vi "DHE_set_roi_transf.vi"(8 "error in (no error)":errorcluster, 10 "args":string) -> (0 "error out":errorcluster, 1 "full":bool, 2 "roi":string, 4 "add roi":bool)   [LabVIEW 2016]
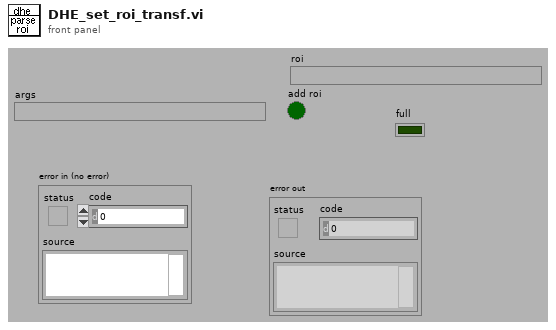
[diagram p1: front panel]
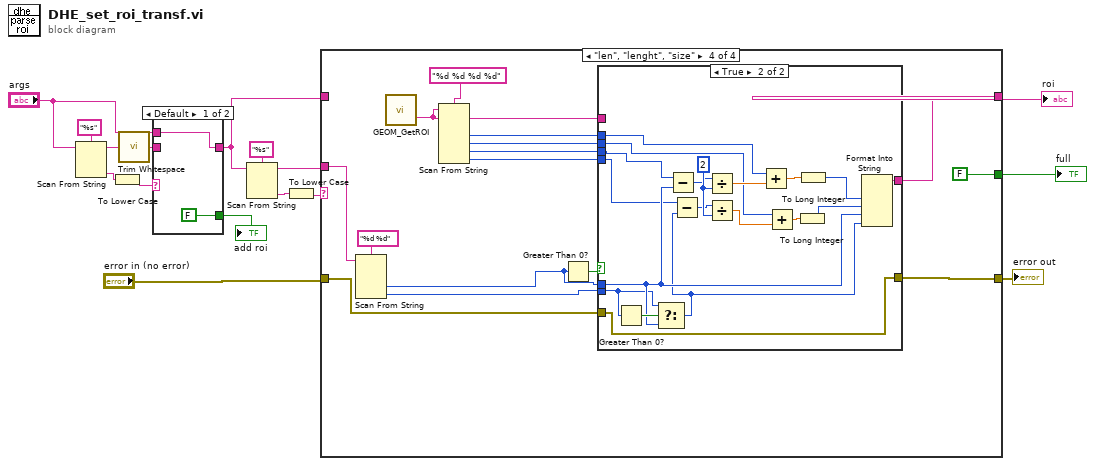
[diagram p0: block diagram]
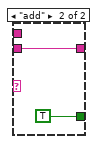
[diagram p2: hidden frame]
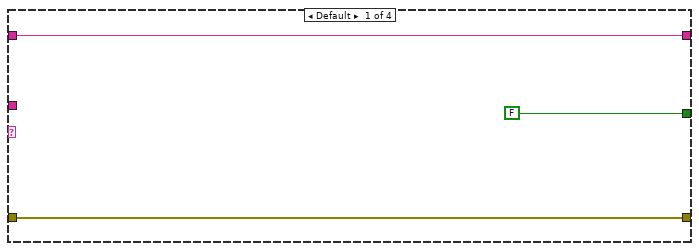
[diagram p3: hidden frame]
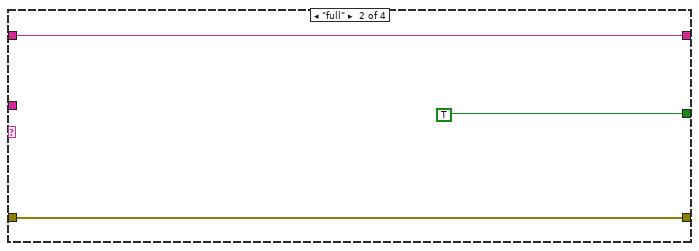
[diagram p4: hidden frame]
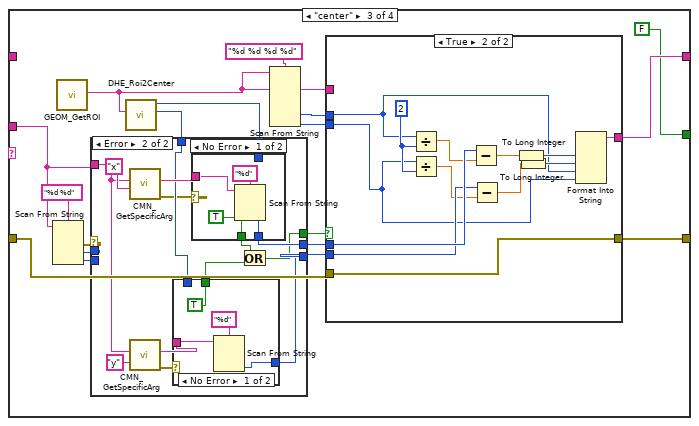
[diagram p5: hidden frame]
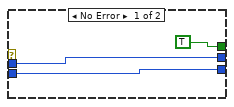
[diagram p6: hidden frame]
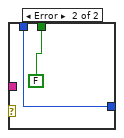
[diagram p7: hidden frame]
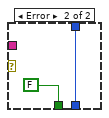
[diagram p8: hidden frame]
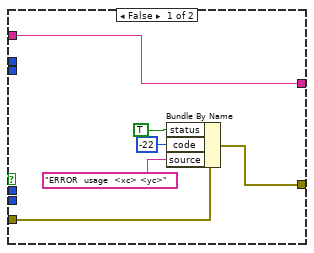
[diagram p9: hidden frame]
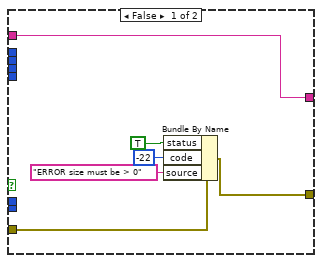
[diagram p10: hidden frame]
diagram:
  n1 = Scan From String(format string="%s", input string="args") -> (remaining string=w5:string, output 1=w7:string)  [unwired: 2 in, 3 out]
  n2 = To Lower Case(string=w7) -> (all lower case string=w6:string)
  n3 = call <vilib>:"Trim Whitespace.vi"("string"=w5) -> ("trimmed string"=w4:string)  [unwired: 1 in]
  n4 = case shown="Default" w6 {
    tunnel: w4 -> [_ w20]
    tunnel: [w18 w20] -> w3
    tunnel: "args" -> [w18 _]
    tunnel: [FALSE TRUE] -> w1
    frame Default {
    }
    frame "add" {
    }
  }
  "add roi" <- w1
  n5 = Scan From String(format string="%s", input string=w3) -> (remaining string=w12:string, output 1=w15:string)  [unwired: 2 in, 3 out]
  n6 = To Lower Case(string=w15) -> (all lower case string=w14:string)
  n7 = case shown="\"len\", \"lenght\", \"size\"" w14 {
    tunnel: w3 -> [w23 w26 _ _]
    tunnel: [w23 w26 w43 w106] -> w13
    tunnel: w12 -> [_ _ w34 w99]
    tunnel: "error in (no error)" -> [w22 w25 w42 w104]
    tunnel: [w22 w25 w41 w103] -> w10
    tunnel: [FALSE ("full") TRUE ("full") FALSE ("full") FALSE ("full")] -> w9
    frame Default {
    }
    frame "full" {
    }
    frame "center" {
      n8 = Scan From String(format string="%d %d", input string=w34) -> (error out=w39:errorcluster, output 1=w38:i32, output 2=w36:i32)  [unwired: 2 in, 4 out]
      n9 = call "GEOM_GetROI.vi"() -> ("Requested ROI"=w30:string)  [unwired: 1 in, 10 out]
      n10 = call "DHE_Roi2Center.vi"("roi"=w30) -> ("yc"=w28:i32, "xc"=w29:i32)  [unwired: 9 out]
      n11 = case shown="Error" w39 {
        tunnel: w38 -> [w47 _]
        tunnel: [w47 w59] -> w37
        tunnel: [w46 w54] -> w35
        tunnel: w36 -> [w46 _]
        tunnel: w34 -> [_ w58]
        tunnel: w29 -> [_ w53]
        tunnel: w28 -> [_ w52]
        tunnel: [TRUE w48] -> w27
        frame No Error {
        }
        frame Error {
          n12 = call "CMN_GetSpecificArg.vi"("key name"="x", "command list"=w58) -> ("error out"=w51:errorcluster, "value"=w60:string)  [unwired: 1 in, 7 out]
          n13 = call "CMN_GetSpecificArg.vi"("key name"="y", "command list"=w58) -> ("error out"=w56:errorcluster, "value"=w55:string)  [unwired: 1 in, 7 out]
          n14 = case shown="No Error" w56 {
            tunnel: w55 -> [w64 _]
            tunnel: [w63 w67] -> w54
            tunnel: w52 -> [_ w67]
            tunnel: [TRUE FALSE] -> w49
            frame No Error {
              n15 = Scan From String(format string="%d", input string=w64) -> (output 1=w63:i32)  [unwired: 2 in, 4 out]
            }
            frame Error {
            }
          }
          n16 = case shown="No Error" w51 {
            tunnel: w60 -> [w71 _]
            tunnel: [w69 w73] -> w59
            tunnel: w53 -> [_ w73]
            tunnel: [TRUE FALSE] -> w50
            frame No Error {
              n17 = Scan From String(format string="%d", input string=w71) -> (output 1=w69:i32)  [unwired: 2 in, 4 out]
            }
            frame Error {
            }
          }
          n18 = Or(x=w50, y=w49) -> (x .or. y?=w48:bool)
        }
      }
      n19 = Scan From String(format string="%d %d %d %d", input string=w30) -> (output 3=w32:i32, output 4=w31:i32)  [unwired: 2 in, 9 out]
      n20 = case shown="True" w27 {
        tunnel: w30 -> [w79 _]
        tunnel: w37 -> [_ w91]
        tunnel: w35 -> [_ w89]
        tunnel: [w79 w87] -> w43
        tunnel: w42 -> [w78 w82]
        tunnel: [w76 w82] -> w41
        tunnel: w32 -> [_ w81]
        tunnel: w31 -> [_ w80]
        frame False {
          n21 = Bundle By Name(cluster=w78, "status"=TRUE, "code"=-22, "source"="ERROR  usage  <xc> <yc>") -> (w76:errorcluster)
        }
        frame True {
          w92 = 2 ("y")
          n22 = Divide(x=w81, y=w92) -> (x/y=w90:dbl)
          n23 = Divide(x=w80, y=w92) -> (x/y=w88:dbl)
          n24 = Subtract(x=w91, y=w90) -> (x-y=w86:dbl)
          n25 = Subtract(x=w89, y=w88) -> (x-y=w85:dbl)
          n26 = To Long Integer(number=w86) -> (32bit integer=w84:i32)
          n27 = To Long Integer(number=w85) -> (32bit integer=w83:i32)
          n28 = Format Into String(w84, w83, w81, w80) -> (resulting string=w87:string)  [unwired: 3 in, 1 out]
        }
      }
    }
    frame "len", "lenght", "size" {
      n29 = Scan From String(format string="%d %d", input string=w99) -> (output 1=w101:i32, output 2=w100:i32)  [unwired: 2 in, 5 out]
      n30 = call "GEOM_GetROI.vi"() -> ("Requested ROI"=w98:string)  [unwired: 1 in, 10 out]
      n31 = Scan From String(format string="%d %d %d %d", input string=w98) -> (output 1=w96:i32, output 2=w95:i32, output 3=w94:i32, output 4=w93:i32)  [unwired: 2 in, 7 out]
      n32 = Greater Than 0?(x=w101) -> (x > 0?=w105:bool)
      n33 = case shown="True" w105 {
        tunnel: w98 -> [w113 _]
        tunnel: [w113 w132] -> w106
        tunnel: w100 -> [_ w119]
        tunnel: w101 -> [_ w120]
        tunnel: w104 -> [w112 w121]
        tunnel: [w111 w121] -> w103
        tunnel: w96 -> [_ w114]
        tunnel: w95 -> [_ w115]
        tunnel: w94 -> [_ w116]
        tunnel: w93 -> [_ w117]
        frame False {
          n34 = Bundle By Name(cluster=w112, "status"=TRUE, "code"=-22, "source"="ERROR size must be > 0") -> (w111:errorcluster)
        }
        frame True {
          w131 = 2 ("y")
          n35 = Greater Than 0?(x=w119) -> (x > 0?=w122:bool)
          n36 = Select(t=w119, s=w122, f=w120) -> (s? t:f=w118:i32)
          n37 = Subtract(x=w116, y=w120) -> (x-y=w124:i32)
          n38 = Subtract(x=w117, y=w118) -> (x-y=w123:i32)
          n39 = Divide(x=w124, y=w131) -> (x/y=w130:dbl)
          n40 = Divide(x=w123, y=w131) -> (x/y=w129:dbl)
          n41 = Add(x=w114, y=w130) -> (x+y=w128:dbl)
          n42 = Add(x=w115, y=w129) -> (x+y=w127:dbl)
          n43 = To Long Integer(number=w127) -> (32bit integer=w126:i32)
          n44 = To Long Integer(number=w128) -> (32bit integer=w125:i32)
          n45 = Format Into String(w125, w126, w120, w118) -> (resulting string=w132:string)  [unwired: 3 in, 1 out]
        }
      }
    }
  }
  "roi" <- w13
  "error out" <- w10
  "full" <- w9
